vi "Create AI Voltage Channel.vi"(8 "error in (no error)":errorcluster, 9 "Physical channel":string, 10 "Name":string, 11 "Task in":refnum<k21>) -> (0 "error out":errorcluster, 2 "Voltage Channel Settings":string, 3 "Task out":refnum<k21>)   [LabVIEW 2021, in "Load Frame.lvlib"]
doc: "Create an AI Voltage channel for 'Physical channel' with 'Name'."
uses:
  Load Frame.lvlib
  <vilib>/DAQmx/create/channels.llb/DAQmx Create Channel (AI-Voltage-Basic).vi
  <resource>/objmgr/daqmx.rc
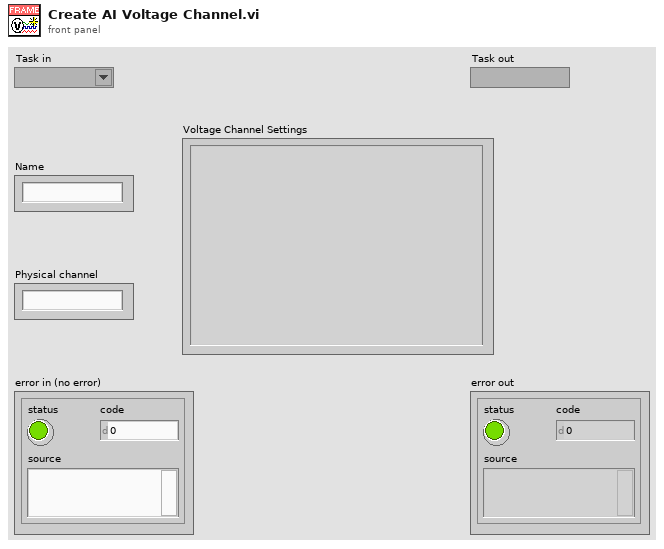
[diagram p1: front panel]
types:
  T1 = cluster{"Name":string, "Physical channel":string, "AI.Max":dbl, "AI.Min":dbl, "AI.MeasType":i32}
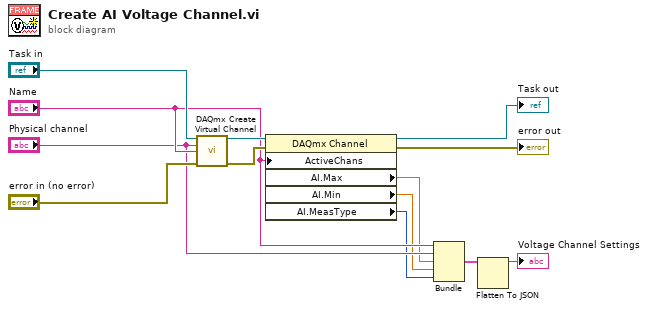
[diagram p0: block diagram]
diagram:
  n1 = call-poly <vilib>:"DAQmx Create Virtual Channel.vi"("task in"="Task in", "physical channels"="Physical channel", "name to assign"="Name", "error in"="error in (no error)") -> ("task out"=w11:refnum<k21>, "error out"=w9:errorcluster)  [unwired: 10 in]
  n2 = property class="DAQmx Channel"(reference=w11, error in=w9, "ActiveChans"="Name") -> (reference out=→"Task out":refnum<k21>, error out=→"error out":errorcluster, "AI.Max"=w5:dbl, "AI.Min"=w4:dbl, "AI.MeasType"=w3:i32)
  n3 = Bundle("Name"="Name", "Physical channel"="Physical channel", "AI.Max"=w5, "AI.Min"=w4, "AI.MeasType"=w3) -> (w1:T1)  [unwired: 1 in]
  n4 = Flatten To JSON(anything=w1) -> (JSON string=→"Voltage Channel Settings":string)  [unwired: 2 in, 1 out]
